vi "PLL_On_Off (SubVI).vi"(8 "error in (no error)":errorcluster, 9 "Output ON/OFF (F=OFF)":bool, 11 "Application in":refnum<vi>) -> (0 "error out":errorcluster, 3 "Application out":refnum<vi>)   [LabVIEW 2014]
uses:
  <userlib>/Nanonis Prog Interface V5/Nanonis Prog Interface.lvlib
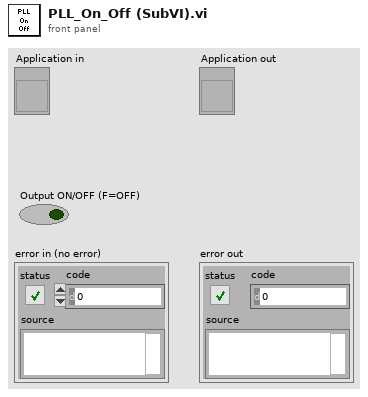
[diagram p1: front panel]
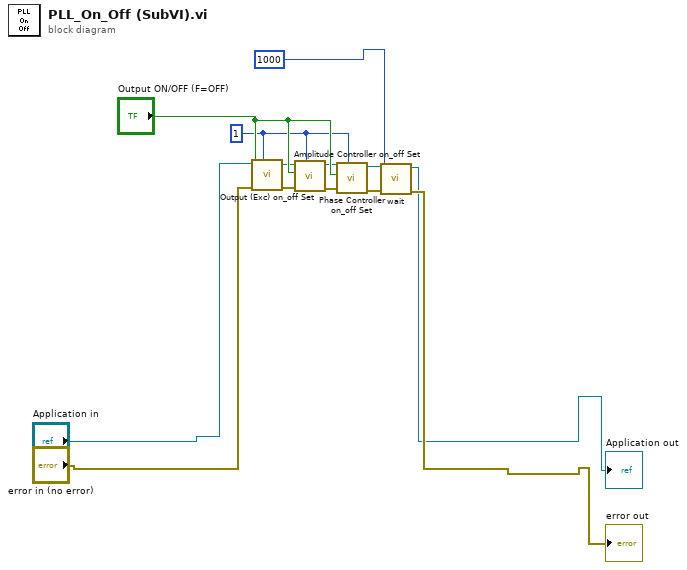
[diagram p0: block diagram]
diagram:
  w6 = 1 ("Modulator index")
  n1 = call <userlib>:"Output (Exc) on_off Set.vi"("Modulator index"=w6, "Error in (no error)"="error in (no error)", "Output ON/OFF (F=OFF)"="Output ON/OFF (F=OFF)", "Application ref in"="Application in") -> ("Error out"=w3:errorcluster, "Application ref out"=w2:refnum<vi>)  [unwired: 6 in]
  n2 = call <userlib>:"Amplitude Controller on_off Set.vi"("Modulator index"=w6, "Error in (no error)"=w3, "Amplitude controller ON/OFF"="Output ON/OFF (F=OFF)", "Application ref in"=w2) -> ("Error out"=w5:errorcluster, "Application ref out"=w4:refnum<vi>)  [unwired: 6 in]
  n3 = call <userlib>:"Phase Controller on_off Set.vi"("Modulator index"=w6, "Error in (no error)"=w5, "Phase controller ON/OFF"="Output ON/OFF (F=OFF)", "Application ref in"=w4) -> ("Error out"=w9:errorcluster, "Application ref out"=w8:refnum<vi>)  [unwired: 6 in]
  n4 = call "wait.vi"("error in"=w9, "milliseconds to wait"=u32 1000 ("y"), "application reference in"=w8) -> ("error out"=→"error out":errorcluster, "application reference out"=→"Application out":refnum<vi>)  [unwired: 7 in]
